vi "Process Chunk.vi"(9 "H In":u32[](array[numeric]), 10 "W In":u32[](array[numeric]), 11 "Chunk":u32[](array[numeric])) -> (1 "H":u32[](array[numeric]), 2 "W":u32[](array[numeric]))   [LabVIEW 2018, in "Crypto.lvlib" / "SHA-256.lvclass"]
uses:
  SHA-256.lvclass
  Temp1.vi
  Temp2.vi
  Sigma1.vi
  Choice.vi
  K.vi
  Sigma0.vi
  Major.vi
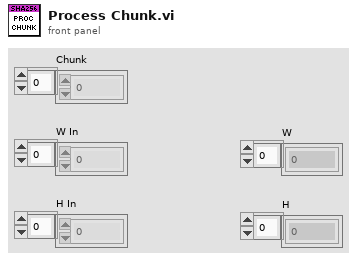
[diagram p1: front panel]
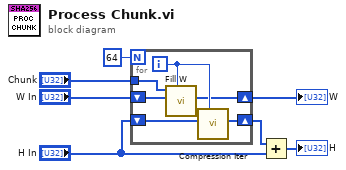
[diagram p0: block diagram]
diagram:
  n1 = for {
    N: 64 -> [_]
    shift-right: [w13] -> w7
    shift-left: "H In" -> [w14]
    shift-right: [w10] -> w2
    shift-left: "W In" -> [w12]
    tunnel: "Chunk" -> [w8]
    i -> [w11]
    n2 = call "Fill W.vi"("i"=w11, "W In"=w12, "Chunk"=w8) -> ("W"=w10:u32[], "W[i]"=w9:u32)  [unwired: 7 in]
    n3 = call "Compression Iter.vi"("i"=w11, "Var In"=w14, "w[i]"=w9) -> ("Var"=w13:u32[])  [unwired: 8 in]
  }
  "W" <- w2
  n4 = Add(x=w7, y="H In") -> (x+y=→"H":u32[])
